vi "Prepare for Close.vi"(8 "error in (no error)":errorcluster, 11 "Application Data in":T1) -> (0 "error out":errorcluster, 2 "file path":path, 3 "Application Data out":T1)   [LabVIEW 2017, in "DSF Configuration Utility.lvlib"]
uses:
  DSF Configuration Utility.lvlib
  Application Data.ctl
  DSF Configuration API/1.0.0/Public/Controls/DSF Config Data RefNum.ctl
  View Mode.ctl
  DSF Configuration API/1.0.0/DSF Configuration API.lvlib
panel:
  # "App\nData"
  # "App\nData"
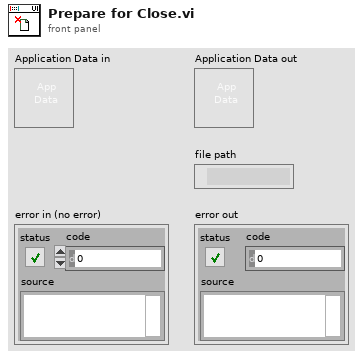
[diagram p1: front panel]
types:
  T1 = typedef "DSF Configuration Utility.lvlib/Application Data.ctl" = cluster{"Item Tree Control":refnum<vi>, "Value Tree Control":refnum<vi>, "DSF Refnum":T2, "Top-Level VI":refnum<vi>, "View State":T3, "menu reference":refnum<k9>}
  T2 = typedef "DSF Configuration API.lvlib/DSF Config Data RefNum.ctl" = refnum<k1>
  T3 = typedef "DSF Configuration Utility.lvlib/View Mode.ctl" = enum16{"Tree", "List"}
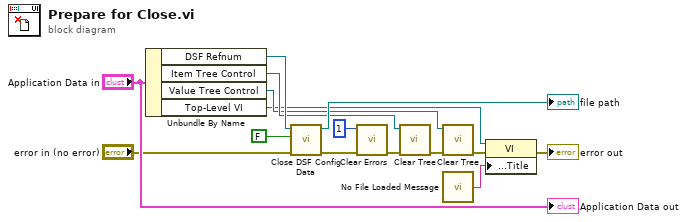
[diagram p0: block diagram]
diagram:
  n1 = Unbundle By Name("Application Data in") -> ("DSF Refnum"=w13:T2, "Item Tree Control"=w6:refnum<vi>, "Value Tree Control"=w5:refnum<vi>, "Top-Level VI"=w4:refnum<vi>)
  n2 = call "Close DSF Config Data.vi"("error in (no error)"="error in (no error)", "write file if changed (T)"=FALSE, "refnum"=w13) -> ("error out"=w12:errorcluster, "file path"=→"file path":path)  [unwired: 7 in]
  n3 = call <vilib>:"Clear Errors.vi"("error in (no error)"=w12, "specific error code to clear (0: all)"=1) -> ("error out"=w8:errorcluster)  [unwired: 4 in, 1 out]
  n4 = call "Clear Tree.vi"("error in (no error)"=w8, "TreeControl in"=w6) -> ("error out"=w7:errorcluster)  [unwired: 9 in]
  n5 = call "Clear Tree.vi"("error in (no error)"=w7, "TreeControl in"=w5) -> ("error out"=w2:errorcluster)  [unwired: 9 in]
  n6 = call "No File Loaded Message.vi"() -> ("no file loaded string"=w3:string)  [unwired: 1 in]
  n7 = property class="VI"(reference=w4, error in=w2, "Front Panel.Title"=w3) -> (error out=→"error out":errorcluster)  [unwired: 1 out]
  "Application Data out" <- "Application Data in"
